vi "CommandPSNumber2 (SubVI).vi"(9 "Storage zone":u8, 11 "data in":string="LON") -> (1 "COMMAND (Hex)":string, 3 "NUMBER":u8)   [LabVIEW 2019, in "SR_2000.lvlib"]
uses:
  SR_2000.lvlib
panel:
  out "type":string
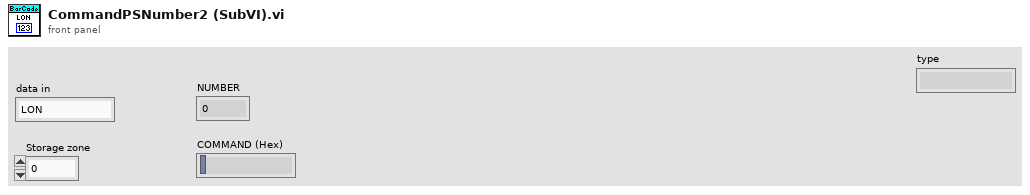
[diagram p1: front panel]
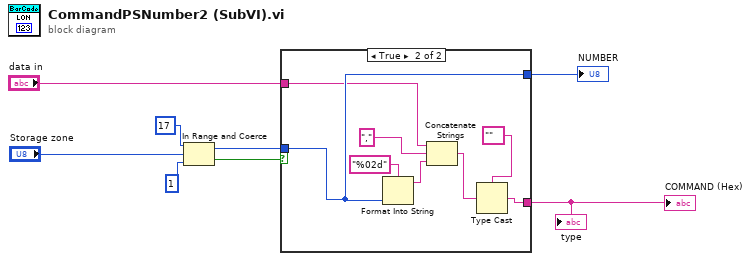
[diagram p0: block diagram]
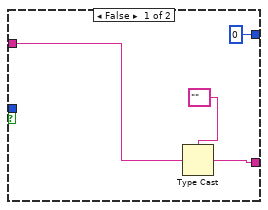
[diagram p2: hidden frame]
diagram:
  n1 = In Range and Coerce(upper limit=u8 17, x="Storage zone", lower limit=u8 1 ("y")) -> (coerced(x)=w8:u8, In Range?=w3:bool)
  n2 = case shown="True" w3 {
    tunnel: [w9 w14] -> w1
    tunnel: w8 -> [_ w18]
    tunnel: [u8 0 ("upper limit") w18] -> w4
    tunnel: "data in" -> [w10 w17]
    frame False {
      n3 = Type Cast(type="", x=w10) -> (*(type *) &x=w9:string)
    }
    frame True {
      n4 = Format Into String(format string="%02d", w18) -> (resulting string=w19:string)  [unwired: 2 in, 1 out]
      n5 = Concatenate Strings(w17, "," ("string"), w19) -> (w15:string)
      n6 = Type Cast(type="", x=w15) -> (*(type *) &x=w14:string)
    }
  }
  "NUMBER" <- w4
  "COMMAND (Hex)" <- w1
  "type" <- w1
